vi "WLAN - niVST - RFSA -Close.vi"(9 "IQ Meas Ref":T1, 10 "Spectrum Meas Ref":T1, 11 "RFSA Handle In":refnum<k15>) -> (0 "error out":errorcluster)   [LabVIEW 2012]
uses:
  <vilib>/RF Toolkits/WLAN/analysis/controls/wlanv1 Analysis Refnum.ctl
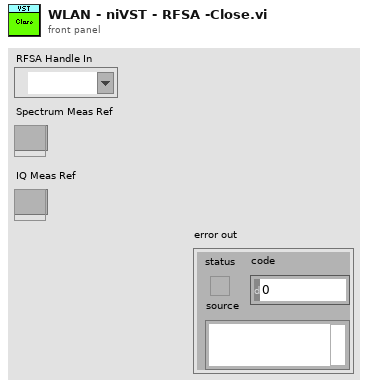
[diagram p1: front panel]
types:
  T1 = typedef "wlanv1 Analysis Refnum.ctl" = refnum<k20>
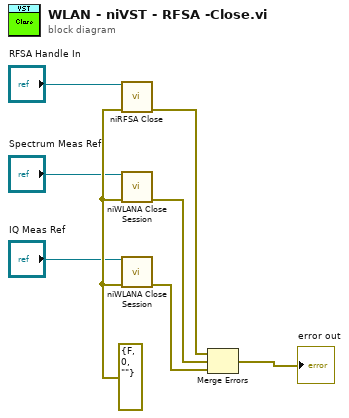
[diagram p0: block diagram]
diagram:
  w7 = errorcluster {"status"=FALSE, "code"=0, "source"=""} ("error in (no error)")
  n1 = call <instrlib>:"niRFSA Close.vi"("instrument handle"="RFSA Handle In", "error in"=w7) -> ("error out"=w4:errorcluster)  [unwired: 13 in]
  n2 = call <vilib>:"niWLANA Close Session.vi"("niwlan analysis session"="Spectrum Meas Ref", "error in"=w7) -> ("error out"=w5:errorcluster)  [unwired: 13 in]
  n3 = call <vilib>:"niWLANA Close Session.vi"("niwlan analysis session"="IQ Meas Ref", "error in"=w7) -> ("error out"=w6:errorcluster)  [unwired: 13 in]
  n4 = Merge Errors(w4, w5, w6) -> (→"error out":errorcluster)
